vi "Disabled.vi"(7 "Robot Mode":T2, 10 "Match Info":T1={"Autonomous Elapsed Seconds"=0.0, "TeleOp Elapsed Seconds"=0.0, "Disabled Elapsed Seconds"=0.0, "Visited Autonomous"=FALSE, "Visited TeleOp"=FALSE, "Visited Disabled"=FALSE, "Autonomous Settings"={"Autonomous Style"=enum."Independent", "VI Refnum"=refnum}}, 11 "Call Context":T3) -> ()   [LabVIEW 2015]
doc: "This VI is called each time a disabled packet is received from the DS. It is often used to prepare for the next robot mode, to calibrate sensors, etc."
uses:
  <vilib>/Rock Robotics/WPI/DriverStation/WPI_DriverStationDerivedRobotMode.ctl
  <vilib>/Rock Robotics/WPI/DriverStation/WPI_DriverStationRobotMode2.ctl
  <vilib>/Rock Robotics/WPI/DriverStation/WPI_DriverStationMatch Info.ctl
  Robot Global Data.vi
  <vilib>/Rock Robotics/Network Tables/SD Read Number.vi
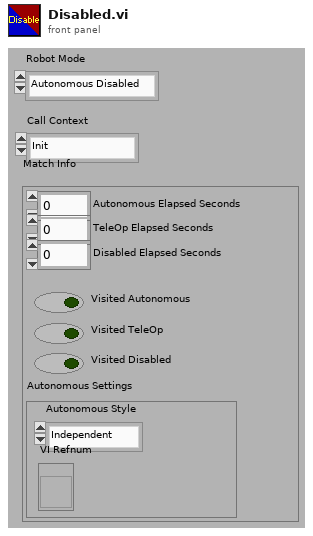
[diagram p1: front panel]
types:
  T1 = typedef "WPI_DriverStationMatch Info.ctl" = cluster{"Autonomous Elapsed Seconds":dbl, "TeleOp Elapsed Seconds":dbl, "Disabled Elapsed Seconds":dbl, "Visited Autonomous":bool, "Visited TeleOp":bool, "Visited Disabled":bool, "Autonomous Settings":cluster{"Autonomous Style":enum16{"Iterative", "Independent"}, "VI Refnum":refnum<vi>}}
  T2 = typedef "WPI_DriverStationRobotMode2.ctl" = enum16{"Autonomous Disabled", "Autonomous Enabled", "Teleop Disabled", "Teleop Enabled", "Disconnected", "Finish", "Test Disabled", "Test Enabled", "Emergency Stopped"}
  T3 = typedef "WPI_DriverStationDerivedRobotMode.ctl" = enum16{"Init", "Execute", "Stop"}
  T4 = typedef "WPI_GyroDevRef.ctl" = cluster{"DevStatus":errorcluster, "Analog Channel":T5, "Offset":dbl, "Gain (VoltsPerDegree/Second)":dbl, "Gyro Type":enum16{"Analog", "XRS450"}, "Handle":i32, "SPI Bus":T6, "Device Found":bool, "Sample Rate":dbl, "Calibrate On Open":bool}
  T5 = typedef "FPGA_AIChannel.ctl" = enum8{"AI 0", "AI 1", "AI 2", "AI 3", "AI MXP 0", "AI MXP 1", "AI MXP 2", "AI MXP 3", "Invalid"}
  T6 = typedef "spi_bus.ctl" = enum16{"SPI On-Board, CS0", "SPI On-Board, CS1", "SPI On-Board, CS2", "SPI On-Board, CS3", "SPI MXP", "Invalid"}
  T7 = typedef "WPI_SwitchDevRef.ctl" = cluster{"DevStatus":errorcluster, "DIO Channel":T8, "CntIndex":T9, "Normally Closed":bool}
  T8 = typedef "FPGA_DIOChannel.ctl" = enum8{"DIO 0", "DIO 1", "DIO 2", "DIO 3", "DIO 4", "DIO 5", "DIO 6", "DIO 7", "DIO 8", "DIO 9", "DIO MXP 0", "DIO MXP 1", "DIO MXP 2", "DIO MXP 3", "DIO MXP 4", "DIO MXP 5", "DIO MXP 6", "DIO MXP 7", "DIO MXP 8", "DIO MXP 9", "DIO MXP 10", "DIO MXP 11", "DIO MXP 12", "DIO MXP 13", "DIO MXP 14", "DIO MXP 15", "Invalid"}
  T9 = typedef "FPGA_CounterCtrSystemIndex.ctl" = enum8{"Ctr 0", "Ctr 1", "Ctr 2", "Ctr 3", "Ctr 4", "Ctr 5", "Ctr 6", "Ctr 7", "Invalid"}
  T10 = typedef "WPI_EncoderDevRef.ctl" = cluster{"DevStatus":errorcluster, "EncoderIndex":T11, "CounterIndex":T9, "DistancePerCount":dbl, "Decoding Type":T12}
  T11 = typedef "FPGA_EncoderIdx.ctl" = enum8{"Enc 0", "Enc 1", "Enc 2", "Enc 3", "Enc 4", "Enc 5", "Enc 6", "Enc 7", "Invalid"}
  T12 = typedef "WPI_EncoderType.ctl" = enum16{"1x", "2x", "4x"}
  T13 = enum16{"No pot 1 bin", "3 Tote Spinny", "2 Tote Middle", "1 Bin", "1 Tote", "Drive", "3 Tote"}
  T14 = typedef "WPI_PotentiometerDevRef.ctl" = cluster{"DevStatus":errorcluster, "Analog Channel":T5, "Invert Output":bool}
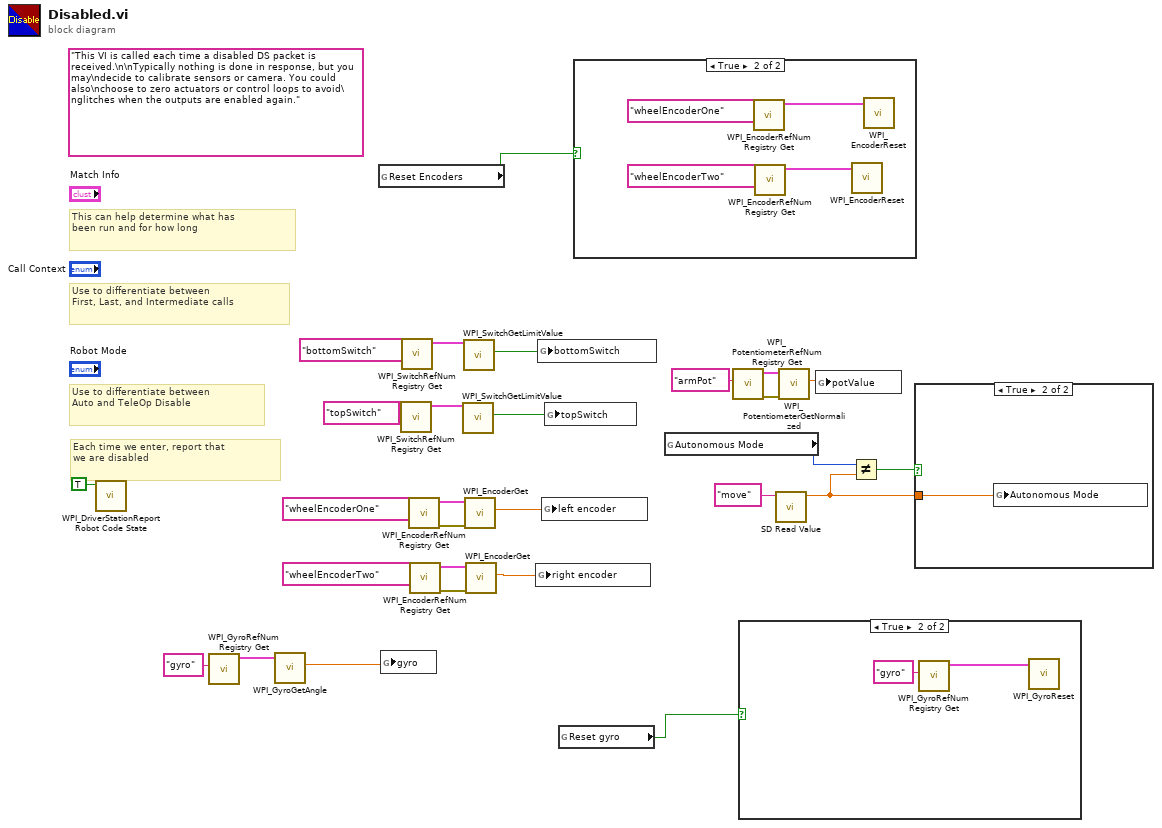
[diagram p0: block diagram]
diagram:
  (unwired) "This VI is called each time a disabled DS packet is received.\n\nTypically nothing is done in response, but you may\ndecide to calibrate sensors or camera. You could also\nchoose to zero actuators or control loops to avoid\nglitches when the outputs are enabled again."
  # "Each time we enter, report that\nwe are disabled"
  # "Use to differentiate between\nFirst, Last, and Intermediate calls"
  # "This can help determine what has\nbeen run and for how long"
  # "Use to differentiate between\nAuto and TeleOp Disable"
  n1 = call <vilib>:"WPI_DriverStationReport Robot Code State.vi"("Disabled"=TRUE ("Autonomous")) -> ()  [unwired: 10 in, 1 out]
  n2 = call <vilib>:"WPI_GyroRefNum Registry Get.vi"("refnum name"="gyro") -> ("GyroDevRef"=w12:T4)  [unwired: 9 in, 1 out]
  n3 = call <vilib>:"WPI_GyroGetAngle.vi"("GyroDevRef"=w12) -> ("Angle"=w11:dbl)  [unwired: 6 in, 4 out]
  n4 = global read "Robot Global Data.vi" "Reset Encoders"() -> (w13:bool)
  n5 = global write "Robot Global Data.vi" "gyro"(w11) -> ()
  n6 = call <vilib>:"WPI_SwitchRefNum Registry Get.vi"("refnum name"="topSwitch") -> ("SwitchDevRef"=w24:T7)  [unwired: 9 in, 1 out]
  n7 = call <vilib>:"WPI_SwitchRefNum Registry Get.vi"("refnum name"="bottomSwitch") -> ("SwitchDevRef"=w27:T7)  [unwired: 9 in, 1 out]
  n8 = call <vilib>:"WPI_EncoderRefNum Registry Get.vi"("refnum name"="wheelEncoderOne") -> ("error out"=w21:errorcluster, "EncoderDevRef"=w20:T10)  [unwired: 9 in]
  n9 = call <vilib>:"WPI_EncoderRefNum Registry Get.vi"("refnum name"="wheelEncoderTwo") -> ("error out"=w18:errorcluster, "EncoderDevRef"=w17:T10)  [unwired: 9 in]
  n10 = call <vilib>:"WPI_SwitchGetLimitValue.vi"("SwitchDevRef"=w24) -> ("Switch Pressed"=w22:bool)  [unwired: 8 in, 2 out]
  n11 = call <vilib>:"WPI_SwitchGetLimitValue.vi"("SwitchDevRef"=w27) -> ("Switch Pressed"=w26:bool)  [unwired: 8 in, 2 out]
  n12 = call <vilib>:"WPI_EncoderGet.vi"("error in (no error)"=w21, "EncoderDevRef"=w20) -> ("Distance"=w15:dbl)  [unwired: 4 in, 5 out]
  n13 = call <vilib>:"WPI_EncoderGet.vi"("error in (no error)"=w18, "EncoderDevRef"=w17) -> ("Distance"=w14:dbl)  [unwired: 4 in, 5 out]
  n14 = global write "Robot Global Data.vi" "right encoder"(w14) -> ()
  n15 = global write "Robot Global Data.vi" "bottomSwitch"(w26) -> ()
  n16 = global write "Robot Global Data.vi" "left encoder"(w15) -> ()
  n17 = global write "Robot Global Data.vi" "topSwitch"(w22) -> ()
  n18 = global read "Robot Global Data.vi" "Reset gyro"() -> (w9:bool)
  n19 = case shown="True" w13 {
    frame False {
    }
    frame True {
      n20 = call <vilib>:"WPI_EncoderRefNum Registry Get.vi"("refnum name"="wheelEncoderOne") -> ("EncoderDevRef"=w30:T10)  [unwired: 9 in, 1 out]
      n21 = call <vilib>:"WPI_EncoderRefNum Registry Get.vi"("refnum name"="wheelEncoderTwo") -> ("EncoderDevRef"=w29:T10)  [unwired: 9 in, 1 out]
      n22 = call <vilib>:"WPI_EncoderReset.vi"("EncoderDevRef"=w29) -> ()  [unwired: 9 in, 2 out]
      n23 = call <vilib>:"WPI_EncoderReset.vi"("EncoderDevRef"=w30) -> ()  [unwired: 9 in, 2 out]
    }
  }
  n24 = global read "Robot Global Data.vi" "Autonomous Mode"() -> (w1:T13)
  n25 = call <vilib>:"WPI_PotentiometerRefNum Registry Get.vi"("refnum name"="armPot") -> ("error out"=w7:errorcluster, "PotDevRef"=w6:T14)  [unwired: 9 in]
  n26 = case shown="True" w9 {
    frame False {
    }
    frame True {
      n27 = call <vilib>:"WPI_GyroRefNum Registry Get.vi"("refnum name"="gyro") -> ("GyroDevRef"=w33:T4)  [unwired: 9 in, 1 out]
      n28 = call <vilib>:"WPI_GyroReset.vi"("GyroDevRef"=w33) -> ()  [unwired: 9 in, 2 out]
    }
  }
  n29 = call-poly <vilib>:"SD Read Value.vi"("Name"="move") -> ("Numeric"=w2:dbl)  [unwired: 8 in, 2 out]
  n30 = call <vilib>:"WPI_PotentiometerGetNormalized.vi"("error in"=w7, "PotDevRef"=w6) -> ("Normalized Value"=w5:dbl)  [unwired: 7 in, 2 out]
  n31 = global write "Robot Global Data.vi" "potValue"(w5) -> ()
  n32 = Not Equal?(x=w1, y=w2) -> (x != y?=w3:bool)
  n33 = case shown="True" w3 {
    tunnel: w2 -> [_ w35]
    frame False {
    }
    frame True {
      n34 = global write "Robot Global Data.vi" "Autonomous Mode"(w35) -> ()
    }
  }
